vi "CEID Manager.vi"(8 "error in (no error)":errorcluster, 11 "S2F37":T2) -> (0 "error out":errorcluster, 3 "S2F38":T1)   [LabVIEW 2020, in "SECS Scenarios.lvlib" / "35-CEID EnableDisable.lvclass"]
uses:
  35-CEID EnableDisable.lvclass
  SECS Communication/S2 Message Class/S2F37.ctl
  SECS Communication/S2 Message Class/S2F38.ctl
  SECS Communication/SECS Data Class/Get CEID Data.vi
  SECS Communication/SECS Data Class/Put CEID Data.vi
  SECS Communication/SECS Data Class/SECS Data Class.lvclass
  SECS Communication/S2 Message Class/S2 Message Class.lvclass
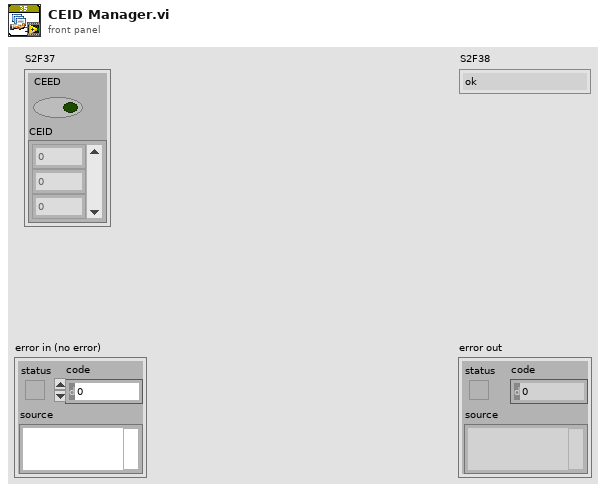
[diagram p1: front panel]
types:
  T1 = typedef "SECS Communication.lvlib/S2 Message Class.lvclass/S2F38.ctl" = enum16{"ok", "denied"}
  T2 = typedef "SECS Communication.lvlib/S2 Message Class.lvclass/S2F37.ctl" = cluster{"CEED":bool, "CEID":u32[]}
  T3 = typedef "SECS Communication.lvlib/SECS Data Class.lvclass/CEID Data.ctl" = cluster{"Enable":bool, "CEID":u32, "Name":string, "Description":string, "RPTID":u32[], "Dynamic":bool}
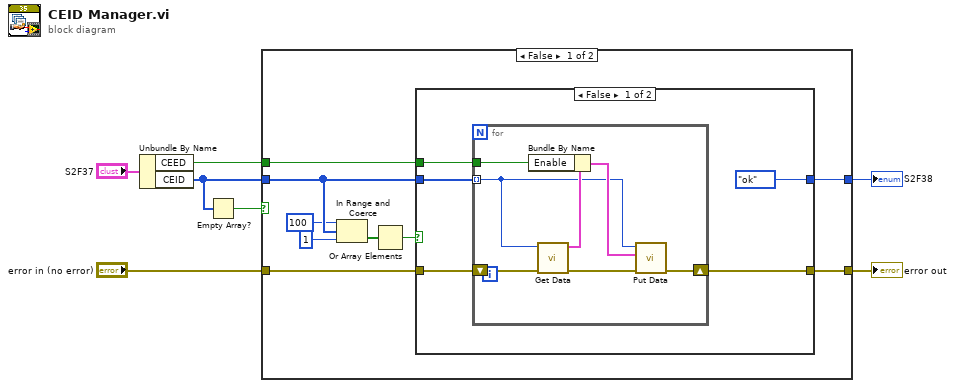
[diagram p0: block diagram]
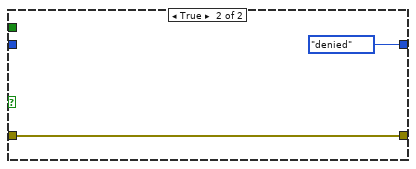
[diagram p2: hidden frame]
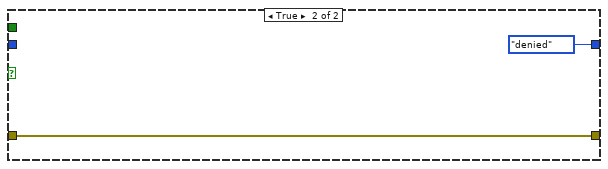
[diagram p3: hidden frame]
diagram:
  n1 = Unbundle By Name("S2F37") -> ("CEED"=w4:bool, "CEID"=w2:u32[])
  n2 = Empty Array?(array=w2) -> (empty?=w1:bool)
  n3 = case shown="False" w1 {
    tunnel: [w16 S2F38."denied" ("S2F38")] -> w6
    tunnel: [w15 w31] -> w5
    tunnel: w4 -> [w14 _]
    tunnel: "error in (no error)" -> [w13 w31]
    tunnel: w2 -> [w12 _]
    frame False {
      n4 = In Range and Coerce(upper limit=u32 100, x=w12, lower limit=u32 1) -> (In Range?=w9:bool[])  [unwired: 1 out]
      n5 = Or Array Elements(Boolean array=w9) -> (logical OR=w8:bool)
      n6 = case shown="False" w8 {
        tunnel: [S2F38."ok" ("S2F38") S2F38."denied" ("S2F38")] -> w16
        tunnel: [w20 w30] -> w15
        tunnel: w14 -> [w17 _]
        tunnel: w13 -> [w19 w30]
        tunnel: w12 -> [w18 _]
        frame False {
          n7 = for {
            shift-right: [w22] -> w20
            shift-left: w19 -> [w28]
            tunnel: w18 -> [w23] mode=indexing
            tunnel: w17 -> [w26]
            n8 = call-poly "Get Data.vi"("error in"=w28, "CEID"=w23) -> ("error out"=w25:errorcluster, "CEID Data"=w27:T3)  [unwired: 7 in, 1 out]
            n9 = Bundle By Name(cluster=w27, "Enable"=w26) -> (w24:T3)
            n10 = call-poly "Put Data.vi"("error in"=w25, "CEID Data"=w24, "CEID"=w23) -> ("error out"=w22:errorcluster)  [unwired: 7 in, 1 out]
          }
        }
        frame True {
        }
      }
    }
    frame True {
    }
  }
  "error out" <- w5
  "S2F38" <- w6
